vi "Write States.vi"(8 "error in (no error)":errorcluster, 10 "States":T1, 11 "DefendGoalTactic in":refnum<class "DefendGoalTactic.lvclass">) -> (0 "error out":errorcluster, 3 "DefendGoalTactic out":refnum<class "DefendGoalTactic.lvclass">)   [LabVIEW 2024, in "DefendGoalTactic.lvclass"]
uses:
  DefendGoalTactic.lvclass
  DefendGoalTacticStates.ctl
  DefendGoalTactic.lvclass/DefendGoalTactic.ctl
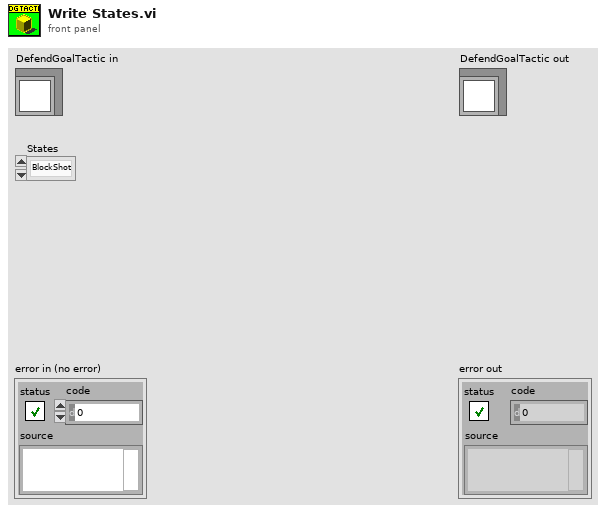
[diagram p1: front panel]
types:
  T1 = typedef "DefendGoalTactic.lvclass/DefendGoalTacticStates.ctl" = enum16{"BlockShot", "BlockPossibleShot", "CoverOneTouchShot", "Kick", "GuardGoal", "Exit"}
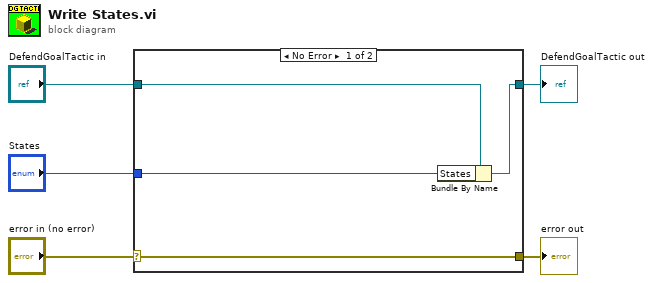
[diagram p0: block diagram]
diagram:
  n1 = case shown="No Error" "error in (no error)" {
    selector: "error in (no error)" -> [w9 w10]
    tunnel: [w9 w10] -> w4
    tunnel: [w7 w11] -> w2
    tunnel: "DefendGoalTactic in" -> [w8 w11]
    tunnel: "States" -> [w6 _]
    frame No Error {
      n2 = Bundle By Name(cluster=w8, "States"=w6) -> (w7:refnum<class "DefendGoalTactic.lvclass">)
    }
    frame Error {
    }
  }
  "error out" <- w4
  "DefendGoalTactic out" <- w2
